vi "SMC Get Witness.vi"() -> (0 "Witness Field":dbl format="%.3f")   [LabVIEW 2010]
uses:
  SMC Global.vi
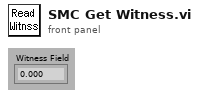
[diagram p1: front panel]
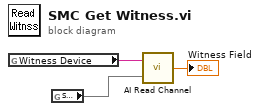
[diagram p0: block diagram]
diagram:
  n1 = global read "SMC Global.vi" "Witness Device"() -> (w2:string)
  n2 = global read "SMC Global.vi" item#-1() -> (w3)
  n3 = call "AI Read Channel.vi"("Channel"=w3, "Device"=w2) -> ("Value"=→"Witness Field":dbl)
